vi "Write Event - New Song.vi"(8 "error in (no error)":errorcluster, 10 "Event - New Song":refnum<user-event>, 11 "SongPlayerActor in":refnum<class "SongPlayerActor.lvclass">) -> (0 "error out":errorcluster, 3 "SongPlayerActor out":refnum<class "SongPlayerActor.lvclass">)   [LabVIEW 2015, in "SongPlayerActor.lvlib" / "SongPlayerActor.lvclass"]
uses:
  SongPlayerActor.lvclass
  file/MusicElement/Song/Song.lvclass
  SongPlayerActor.lvclass/SongPlayerActor.ctl
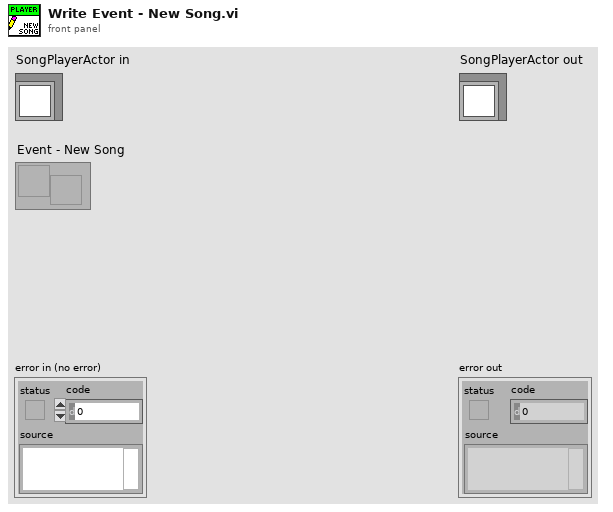
[diagram p1: front panel]
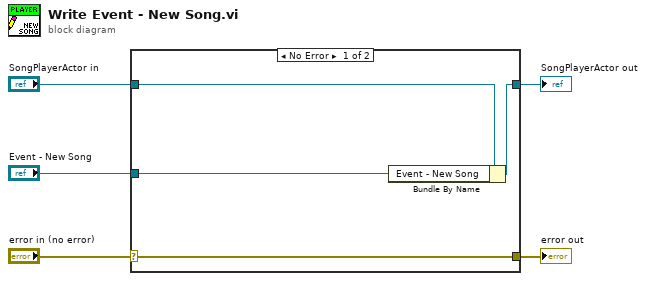
[diagram p0: block diagram]
diagram:
  n1 = case shown="No Error" "error in (no error)" {
    selector: "error in (no error)" -> [w9 w10]
    tunnel: [w9 w10] -> w4
    tunnel: [w7 w11] -> w2
    tunnel: "SongPlayerActor in" -> [w8 w11]
    tunnel: "Event - New Song" -> [w6 _]
    frame No Error {
      n2 = Bundle By Name(cluster=w8, "Event - New Song"=w6) -> (w7:refnum<class "SongPlayerActor.lvclass">)
    }
    frame Error {
    }
  }
  "error out" <- w4
  "SongPlayerActor out" <- w2
